vi "sub vi - AI USB4704 (3) v6.vi"() -> (1 "Graph 1":dynamicdata(graph), 2 "Graph 2":dynamicdata(graph), 3 "Graph 3":dynamicdata(graph), 10 "loop time":dbl format="%.6g", 15 "error array":errorcluster[](array[cluster]))   [LabVIEW 2013]
panel:
  in  "Tab Control":enum32{"Page 1", "Page 2", "Page 3"}(tab)
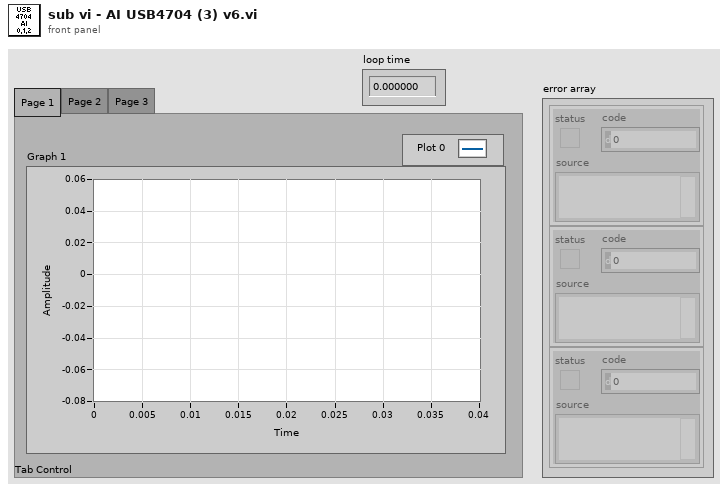
[diagram p1: front panel]
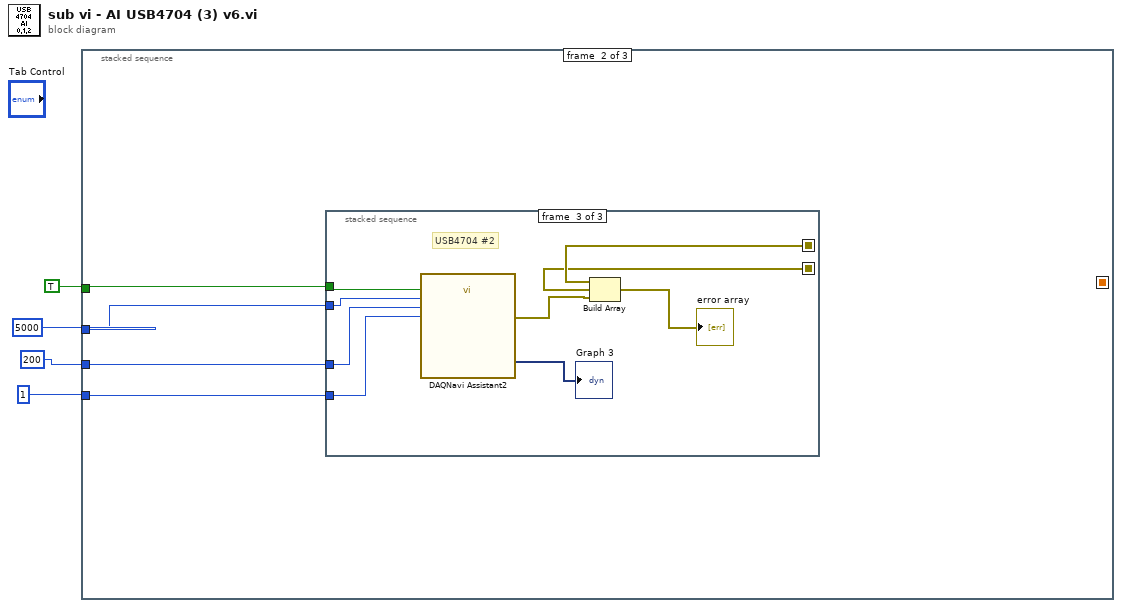
[diagram p0: block diagram]
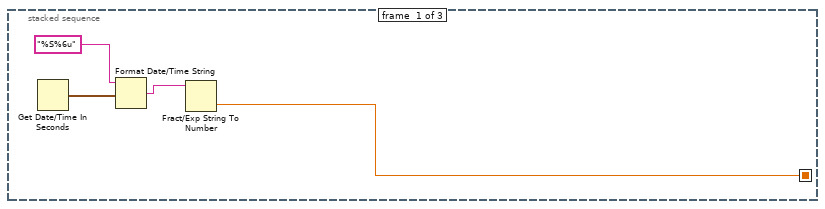
[diagram p2: hidden frame]
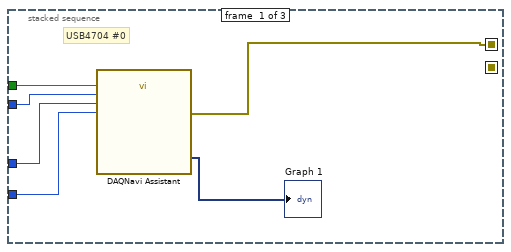
[diagram p3: hidden frame]
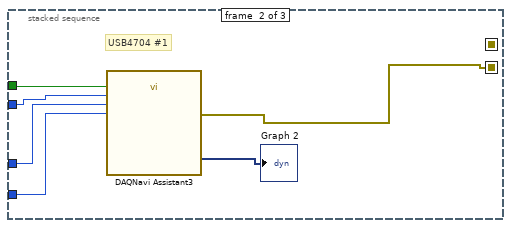
[diagram p4: hidden frame]
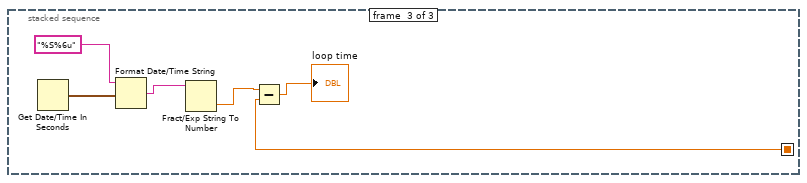
[diagram p5: hidden frame]
diagram:
  n1 = stacked-sequence {
    seq-local: [w5 _ _] -> [_ _ w35]
    tunnel: TRUE -> [_ w12 _]
    tunnel: 1 -> [_ w9 _]
    tunnel: 5000 -> [_ w11 _]
    tunnel: 200 -> [_ w10 _]
    frame #0 {
      n2 = Get Date/Time In Seconds() -> (seconds since 1Jan1904=w7:timestamp)
      n3 = Format Date/Time String(time format string (%c)="%S%6u", seconds (now)=w7) -> (date/time string=w6:string)  [unwired: 1 in]
      n4 = Fract/Exp String To Number(string=w6) -> (number=w5:dbl)  [unwired: 3 in, 1 out]
    }
    frame #1 {
      n5 = stacked-sequence {
        seq-local: [w13 _ _] -> [_ _ w28]
        seq-local: [_ w19 _] -> [_ _ w27]
        tunnel: w12 -> [w17 w24 w33]
        tunnel: w11 -> [w16 w23 w32]
        tunnel: w10 -> [w15 w22 w31]
        tunnel: w9 -> [w14 w21 w30]
        frame #0 {
          # "USB4704 #0"
          n6 = call "DAQNavi Assistant"("stop(true)"=w17, "conversion rate(Hz)"=w16, "samples"=w15, "time out(10s)"=w14) -> ("error out"=w13:errorcluster, "data out(DDT)"=→"Graph 1":dynamicdata)  [unwired: 22 in]
        }
        frame #1 {
          # "USB4704 #1"
          n7 = call "DAQNavi Assistant3"("stop(true)"=w24, "conversion rate(Hz)"=w23, "samples"=w22, "time out(10s)"=w21) -> ("error out"=w19:errorcluster, "data out(DDT)"=→"Graph 2":dynamicdata)  [unwired: 22 in]
        }
        frame #2 {
          # "USB4704 #2"
          n8 = call "DAQNavi Assistant2"("stop(true)"=w33, "conversion rate(Hz)"=w32, "samples"=w31, "time out(10s)"=w30) -> ("error out"=w26:errorcluster, "data out(DDT)"=→"Graph 3":dynamicdata)  [unwired: 22 in]
          n9 = Build Array(w28, w27, w26) -> (→"error array":errorcluster[])
        }
      }
    }
    frame #2 {
      n10 = Get Date/Time In Seconds() -> (seconds since 1Jan1904=w38:timestamp)
      n11 = Format Date/Time String(time format string (%c)="%S%6u", seconds (now)=w38) -> (date/time string=w37:string)  [unwired: 1 in]
      n12 = Fract/Exp String To Number(string=w37) -> (number=w36:dbl)  [unwired: 3 in, 1 out]
      n13 = Subtract(x=w36, y=w35) -> (x-y=→"loop time":dbl)
    }
  }
